vi "Codec_CMD_6.vi"(8 "error in (no error)":errorcluster, 10 "AskCMD6":T1={"STATION"="F/T-B", "RACK"="101", "SN"="AP32023099", "RESULT"=""}, 11 "SecureMqttCodec in":refnum<class "SecureMqttCodec.lvclass">) -> (0 "error out":errorcluster, 2 "<JSON>":string="{\r  \"CMD\": 6,\r  \"CONTENT\": [\r    {\r      \"RACK\": \"101\",\r      \"SN\": \"AP32023099\",\r      \"STATION\": \"F/T-B\"\r    }\r  ],\r  \"ERRCODE\": \"\",\r  \"ERRMSG\": \"\",\r  \"FROM\": \"845CF3525B43\",\r  \"ID\": \"8AAF833C-EF26-463F-96A7-49A13DD312CD\",\r  \"STATUS\": \"\",\r  \"TIMESTAMP\": 1759590678,\r  \"TO\": \"\"\r}", 3 "SecureMqttCodec out":refnum<class "SecureMqttCodec.lvclass">)   [LabVIEW 2020, in "SecureMqttCodec.lvclass"]
uses:
  SecureMqttCodec.lvclass
  TestMQTT/Ctrl/ReplyCMD6.ctl
  SecureMqttCodec.lvclass/SecureMqttCodec.ctl
  <vilib>/addons/JSON API/JSON Value/Set from JSON string.vi
  <vilib>/addons/JSON API/JSON Scalar/JSON Scalar.lvclass
  C:/Program Files/National Instruments/LabVIEW 2020/vi.lib/addons/JSON API/JSON Value/JSON Value.lvclass
  <vilib>/addons/JSON API/JSON Array/JSON Array.lvclass
  <vilib>/addons/JSON API/JSON Scalar/Set U32.vi
  <vilib>/addons/JSON API/JSON Array/Set JSON Array.vi
  <vilib>/addons/JSON API/JSON Value/Get as JSON string (pretty).vi
  <vilib>/addons/JSON API/JSON Value/JSON Value.lvclass
  <vilib>/addons/JSON API/Get Polymorphic/JSON GetSet.lvlib
  <vilib>/addons/JSON API/JSON Object/JSON Object.lvclass
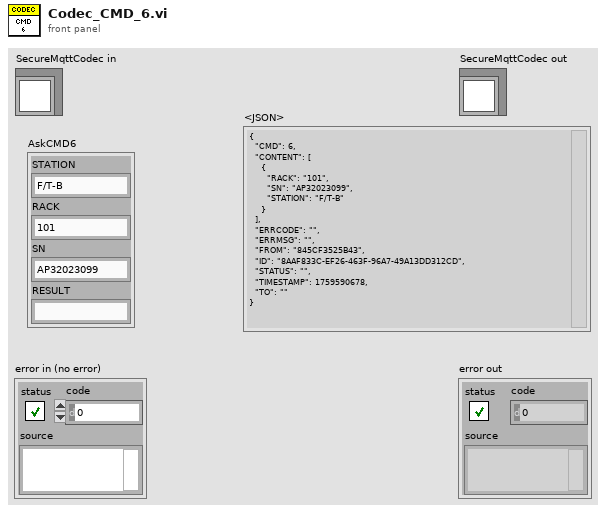
[diagram p1: front panel]
types:
  T1 = typedef "ReplyCMD6.ctl" = cluster{"STATION":string, "RACK":string, "SN":string, "RESULT":string}
  T2 = cluster{"STATION":string, "RACK":string, "SN":string}
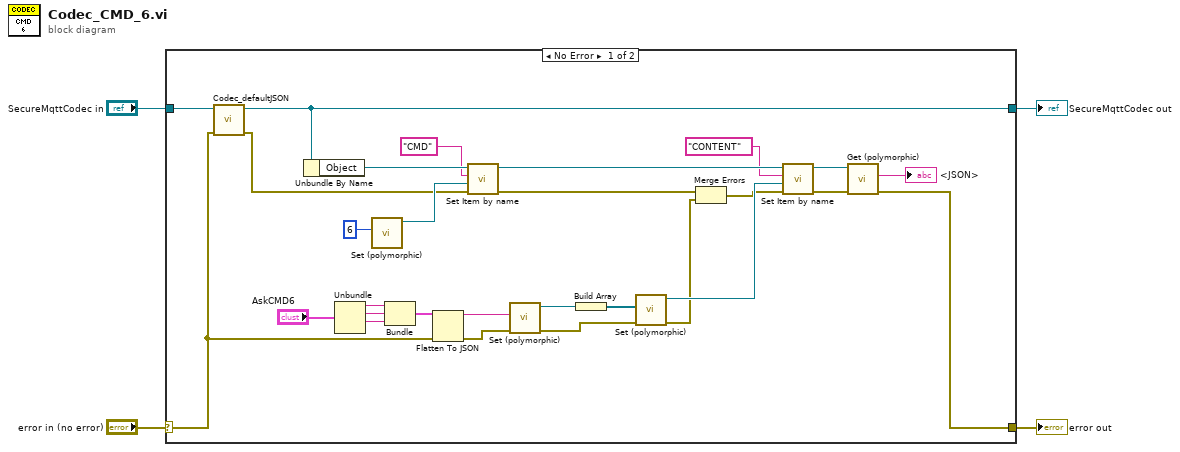
[diagram p0: block diagram]
diagram:
  n1 = case shown="No Error" "error in (no error)" {
    selector: "error in (no error)" -> [w13 w34]
    tunnel: [w28 w34] -> w3
    tunnel: [w20 w33] -> w1
    tunnel: "SecureMqttCodec in" -> [w32 w33]
    frame No Error {
      n2 = call "Codec_defaultJSON.vi"("error in (no error)"=w13, "SecureMqttCodec in"=w32) -> ("error out"=w19:errorcluster, "SecureMqttCodec out"=w20:refnum<class "SecureMqttCodec.lvclass">)  [unwired: 8 in]
      n3 = Unbundle By Name(w20) -> ("Object"=w31:refnum<class "JSON Value.lvclass">)
      n4 = Unbundle("AskCMD6") -> ("STATION"=w9:string, "RACK"=w6:string, "SN"=w5:string)  [unwired: 1 out]
      n5 = call-poly <vilib>:"Set (polymorphic).vi"("Numeric"=u32 6) -> ("JSON Scalar out"=w29:refnum<class "JSON Scalar.lvclass">)  [unwired: 9 in, 1 out]
      n6 = Bundle("STATION"=w9, "RACK"=w6, "SN"=w5) -> (w7:T2)  [unwired: 1 in]
      n7 = Flatten To JSON(anything=w7, error in (no error)=w13) -> (JSON string=w15:string, 11:w14:errorcluster)  [unwired: 1 in]
      n8 = call-dynamic "Set Item by name.vi"("error in (no error)"=w19, "Value"=w29, "name"="CMD", "JSON Value In"=w31) -> ("error out"=w24:errorcluster, "JSON Value Out"=w26:refnum<class "JSON Value.lvclass">)  [unwired: 5 in, 1 out]
      n9 = call-poly <vilib>:"Set (polymorphic).vi"("error in (no error)"=w14, "JSON stream"=w15) -> ("error out"=w12:errorcluster, "JSON Value out"=w17:refnum<class "JSON Value.lvclass">)  [unwired: 7 in, 1 out]
      n10 = Build Array(w17) -> (w16:refnum<class "JSON Value.lvclass">[])
      n11 = call-poly <vilib>:"Set (polymorphic).vi"("error in (no error)"=w12, "Array"=w16) -> ("error out"=w10:errorcluster, "JSON Array out"=w22:refnum<class "JSON Array.lvclass">)  [unwired: 8 in]
      n12 = Merge Errors(w24, w10) -> (w11:errorcluster)
      n13 = call-dynamic "Set Item by name.vi"("error in (no error)"=w11, "Value"=w22, "name"="CONTENT", "JSON Value In"=w26) -> ("error out"=w23:errorcluster, "JSON Value Out"=w25:refnum<class "JSON Value.lvclass">)  [unwired: 5 in, 1 out]
      n14 = call-poly <vilib>:"Get (polymorphic).vi"("error in (no error)"=w23, "JSON Value in"=w25) -> ("error out"=w28:errorcluster, "<JSON>"=→"<JSON>":string)  [unwired: 8 in]
    }
    frame Error {
    }
  }
  "error out" <- w3
  "SecureMqttCodec out" <- w1
